vi "Send Message to Create Child Object.vi"(8 "Error In":errorcluster, 9 "ID of Node to Add To":string, 10 "node type":string, 11 "Queue in":T1) -> (0 "Error Out":errorcluster, 3 "Queue Out":T1)   [LabVIEW 2019, in "Configuration Tool.lvlib"]
doc: "Sends a message to add a node"
uses:
  Configuration Tool.lvlib
  <vilib>/NI/AMC/Message Queue.ctl
  <vilib>/NI/AMC/Message.ctl
  <vilib>/NI/Tools/Keyed Array/KeyedArray.ctl
  Controls/AddMessage.ctl
  <vilib>/NI/AMC/Create Single Message.vi
  <vilib>/NI/AMC/Update Message Routing Info.vi
  <vilib>/NI/AMC/Send Message.vi
  <vilib>/NI/AMC/AMC.lvlib
  <vilib>/NI/Tools/Keyed Array/Tools_KeyedArray.lvlib
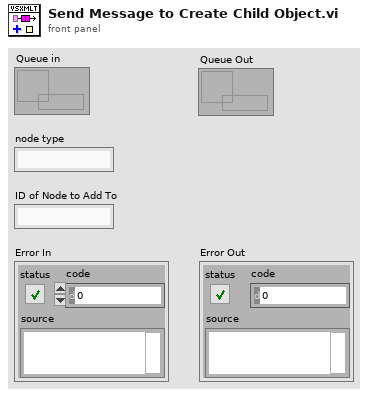
[diagram p1: front panel]
types:
  T1 = typedef "AMC.lvlib/Message Queue.ctl" = refnum<queue>
  T2 = typedef "Configuration Tool.lvlib/AddMessage.ctl" = cluster{"node type":string, "to add to":string}
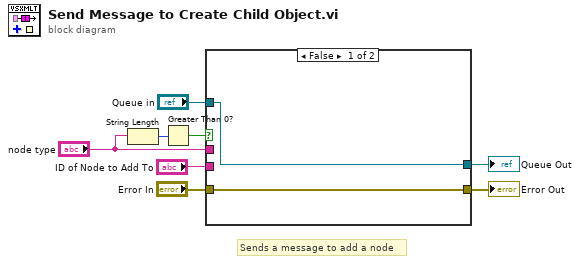
[diagram p0: block diagram]
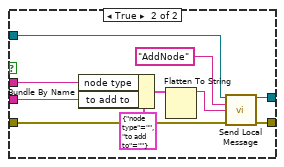
[diagram p2: hidden frame]
diagram:
  # "Sends a message to add a node"
  n1 = String Length(string="node type") -> (length=w4:i32)
  n2 = Greater Than 0?(x=w4) -> (x > 0?=w3:bool)
  n3 = case shown="False" w3 {
    tunnel: "Error In" -> [w10 w16]
    tunnel: [w10 w15] -> w6
    tunnel: "node type" -> [_ w14]
    tunnel: "ID of Node to Add To" -> [_ w13]
    tunnel: "Queue in" -> [w9 w12]
    tunnel: [w9 w11] -> w1
    frame False {
    }
    frame True {
      n4 = Bundle By Name(cluster=T2 {"node type"="", "to add to"=""} ("input cluster"), "node type"=w14, "to add to"=w13) -> (w18:T2)
      n5 = Flatten To String(anything=w18) -> (data string=w19:string)  [unwired: 3 in, 2 out]
      n6 = call <vilib>:"Send Local Message.vi"("message queue in"=w12, "message name"="AddNode" ("Message Name"), "message value"=w19, "error in"=w16) -> ("message queue out"=w11:T1, "error out"=w15:errorcluster)  [unwired: 9 in, 1 out]
    }
  }
  "Error Out" <- w6
  "Queue Out" <- w1
